vi "Read JSON Config.vi"(8 "error in (no error)":errorcluster, 10 "JSON Config":string, 11 "AbsFunc_One Term_U16 in":refnum<class "AbsFunc_One Term_U16.lvclass">) -> (0 "error out":errorcluster, 3 "AbsFunc_One Term_U16 out":refnum<class "AbsFunc_One Term_U16.lvclass">)   [LabVIEW 2021, in "AbsFunc_One Term_U16.lvclass"]
uses:
  AbsFunc_One Term_U16.lvclass
  AbsFunc_One Term_U16.lvclass/AbsFunc_One Term_U16.ctl
  Abs_Types/Type/Abs_Type.lvclass
  Abs_Types/U16 Integer/Abs_U16 Integer.lvclass
  C:/Users/Tim/Documents/GitHub/LV_Abstract/Source/Abs_Types/U16 Integer/Abs_U16 Integer.lvclass
  C:/Users/Tim/Documents/GitHub/LV_Abstract/Source/Abs_Types/Integer/Abs_Integer.lvclass
  C:/Users/Tim/Documents/GitHub/LV_Abstract/Source/Abs_Types/Numeric/Abs_Numeric.lvclass
  C:/Users/Tim/Documents/GitHub/LV_Abstract/Source/Abs_Types/Value/Abs_Value.lvclass
  C:/Users/Tim/Documents/GitHub/LV_Abstract/Source/Abs_Types/Type/Abs_Type.lvclass
  C:/Users/Tim/Documents/GitHub/LV_Abstract/Source/Functions/Support/One Terminal/U16/AbsFunc_One Term_U16.lvclass
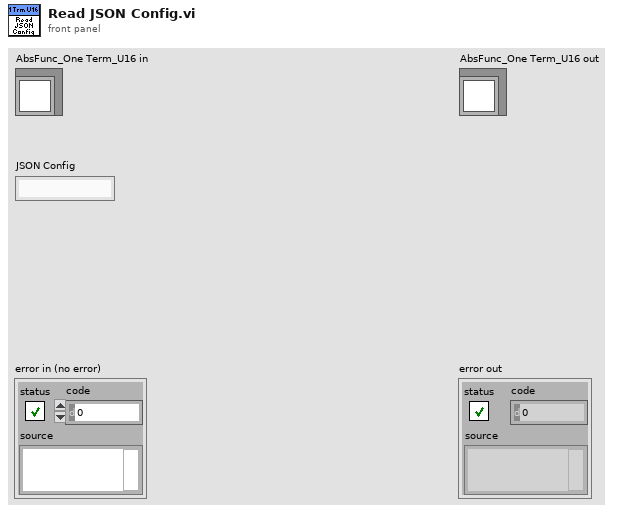
[diagram p1: front panel]
types:
  T1 = typedef "AbsFunc_One Term_U16.lvclass/Abstract Type.ctl" = refnum<class "Abs_U16 Integer.lvclass">
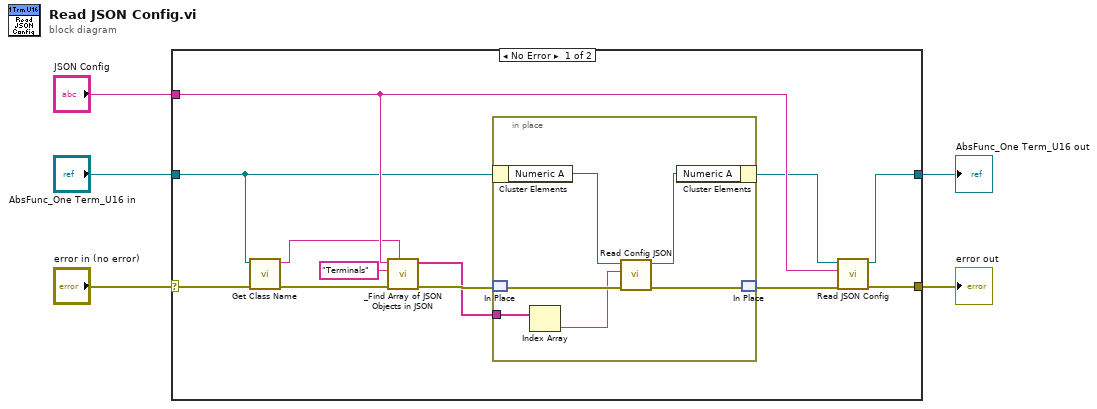
[diagram p0: block diagram]
diagram:
  n1 = case shown="No Error" "error in (no error)" {
    selector: "error in (no error)" -> [w13 w24]
    tunnel: [w17 w24] -> w4
    tunnel: [w16 w25] -> w3
    tunnel: "JSON Config" -> [w15 _]
    tunnel: "AbsFunc_One Term_U16 in" -> [w12 w25]
    frame No Error {
      n2 = call "Get Class Name.vi"("error in (no error)"=w13, "Abs_Type in"=w12) -> ("error out"=w14:errorcluster, "class name"=w7:string)  [unwired: 8 in]
      n3 = call "_Find Array of JSON Objects in JSON.vi"("JSON Object Name"=w7, "error in (no error)"=w14, "JSON Array Name"="Terminals", "JSON Config"=w15) -> ("error out"=w11:errorcluster, "JSON Objects"=w10:string[])  [unwired: 6 in]
      n4 = in-place {
        in-place-border: w10 -> [w23]
        n5 = in-place-cluster #1(w12) -> ("Numeric A"=w19:T1)
        n6 = in-place-match #2(w11) -> (w22:errorcluster)
        n7 = Index Array(array=w23) -> (element=w21:string)  [unwired: 1 in]
        n8 = call "Read Config JSON.vi"("error in (no error)"=w22, "JSON Config"=w21, "Abs_Type in"=w19) -> ("error out"=w20:errorcluster, "Abs_Type out"=w18:T1)  [unwired: 7 in]
        n9 = in-place-cluster #1("Numeric A"=w18) -> (w8:refnum<class "AbsFunc_One Term_U16.lvclass">)
        n10 = in-place-match #2(w20) -> (w9:errorcluster)
      }
      n11 = call-parent "Read JSON Config.vi"("error in (no error)"=w9, "JSON Config"=w15, "Abs_Type in"=w8) -> ("error out"=w17:errorcluster, "Abs_Type out"=w16:refnum<class "AbsFunc_One Term_U16.lvclass">)  [unwired: 7 in]
    }
    frame Error {
    }
  }
  "error out" <- w4
  "AbsFunc_One Term_U16 out" <- w3
